vi "mb Convert [I32] to [U16].vi"(4 "I32":i32, 5 "I32 [ ]":i32[](array[numeric])) -> (1 "U16 [ ]":u16[](array[numeric]))   [LabVIEW 2011]
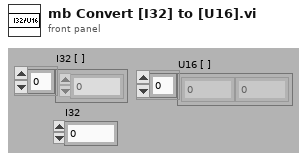
[diagram p1: front panel]
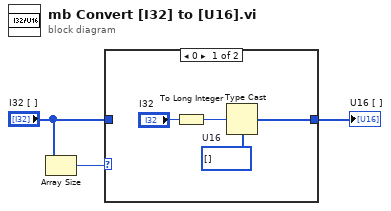
[diagram p0: block diagram]
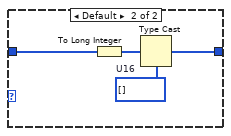
[diagram p2: hidden frame]
diagram:
  n1 = Array Size(array="I32 [ ]") -> (size(s)=w2:i32)
  n2 = case shown="0" w2 {
    tunnel: "I32 [ ]" -> [_ w11]
    tunnel: [w4 w8] -> w1
    frame 0 {
      w6 = u16[] []  # U16
      n3 = To Long Integer(number="I32") -> (32bit integer=w7:i32)
      n4 = Type Cast(type=w6, x=w7) -> (*(type *) &x=w4:u16[])
    }
    frame Default {
      w9 = u16[] []  # U16
      n5 = To Long Integer(number=w11) -> (32bit integer=w10:i32[])
      n6 = Type Cast(type=w9, x=w10) -> (*(type *) &x=w8:u16[])
    }
  }
  "U16 [ ]" <- w1
